vi "Signal Parameters FG.vi"(7 "Action":T1, 8 "error in (no error)":errorcluster, 10 "Signal Parameters":T2 {"Byte Order" items=["Little Endian", "Big Endian"]; "Data Type" items=["Signed", "Unsigned", "IEEE Float"]}, 11 "Device Item Ref in":T3 format="%.0x") -> (0 "error out":errorcluster, 2 "Signal Parameters":T2 {"Byte Order" items=["Little Endian", "Big Endian"]; "Data Type" items=["Signed", "Unsigned", "IEEE Float"]}, 3 "Device Item Ref out":T3=18446744073709551615 format="%.0x")   [LabVIEW 2013, in "Diagnostics Addon Shared.lvlib"]
uses:
  Diagnostics Addon Shared.lvlib
  <vilib>/NI Veristand/Custom Device API/Custom Device Item Ref.ctl
  DIDPID Signal Parameters.ctl
  FG Action.ctl
  GUID Lookup.vi
  <vilib>/NI Veristand/Custom Device API/Set Item Property (Variant).vi
  <vilib>/NI Veristand/Custom Device API/Get Item Property (Variant).vi
  <vilib>/NI Veristand/Custom Device API/Custom Device API.lvlib
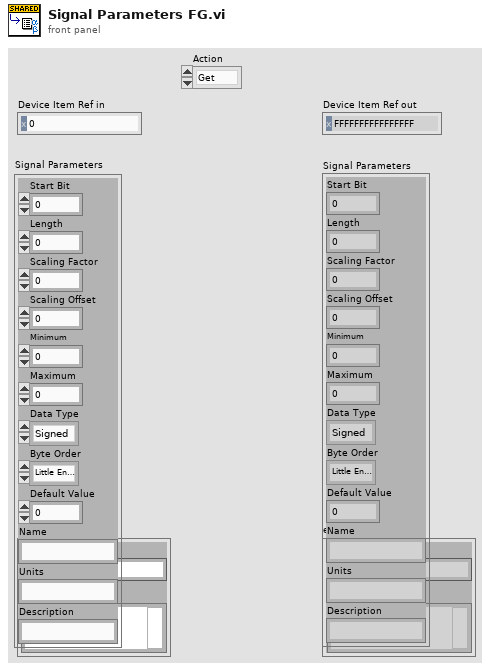
[diagram p1: front panel]
types:
  T1 = typedef "Diagnostics Addon Shared.lvlib/FG Action.ctl" = enum16{"Get", "Set"}
  T2 = typedef "Diagnostics Addon Shared.lvlib/DIDPID Signal Parameters.ctl" = cluster{"Start Bit":u8, "Length":u8, "Scaling Factor":dbl, "Scaling Offset":dbl, "Minimum":dbl, "Maximum":dbl, "Data Type":u32, "Byte Order":u32, "Default Value":dbl, "Name":string, "Units":string, "Description":string}
  T3 = typedef "Custom Device API.lvlib/Custom Device Item Ref.ctl" = u64
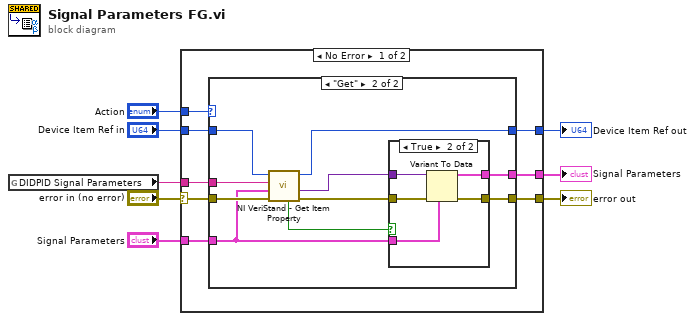
[diagram p0: block diagram]
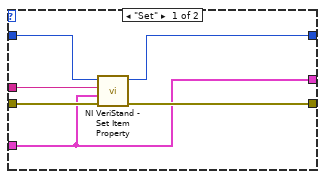
[diagram p2: hidden frame]
diagram:
  n1 = global read "GUID Lookup.vi" "DIDPID Signal Parameters"() -> (w3:string)
  n2 = case shown="No Error" "error in (no error)" {
    selector: "error in (no error)" -> [w16 w40]
    tunnel: "Device Item Ref in" -> [w15 w41]
    tunnel: [w14 w41] -> w5
    tunnel: [w13 w40] -> w6
    tunnel: [w12 _] -> w4
    tunnel: w3 -> [w11 _]
    tunnel: "Signal Parameters" -> [w10 _]
    tunnel: "Action" -> [w9 _]
    frame No Error {
      n3 = case shown="\"Get\"" w9 {
        tunnel: w16 -> [w22 w32]
        tunnel: w15 -> [w18 w31]
        tunnel: [w17 w30] -> w14
        tunnel: [w21 w28] -> w13
        tunnel: [w20 w26] -> w12
        tunnel: w11 -> [w19 w25]
        tunnel: w10 -> [w20 w24]
        frame "Set" {
          n4 = call-poly <vilib>:"NI VeriStand - Set Item Property.vi"("error in (no error)"=w22, "Value"=w20, "Property Name"=w19, "Item Ref in"=w18) -> ("error out"=w21:errorcluster, "Item Ref out"=w17:T3)  [unwired: 5 in, 1 out]
        }
        frame "Get" {
          n5 = call-poly <vilib>:"NI VeriStand - Get Item Property.vi"("error in (no error)"=w32, "Default Value"=w24, "Property Name"=w25, "Item Ref in"=w31) -> ("error out"=w29:errorcluster, "Value"=w27:variant, "Item Ref out"=w30:T3, "Found?"=w23:bool)  [unwired: 4 in]
          n6 = case shown="True" w23 {
            tunnel: w29 -> [w33 w39]
            tunnel: [w33 w38] -> w28
            tunnel: w27 -> [_ w37]
            tunnel: [w34 w36] -> w26
            tunnel: w24 -> [w34 w35]
            frame False {
            }
            frame True {
              n7 = Variant To Data(error in=w39, type=w35, Variant=w37) -> (data=w36:T2, error out=w38:errorcluster)
            }
          }
        }
      }
    }
    frame Error {
    }
  }
  "error out" <- w6
  "Device Item Ref out" <- w5
  "Signal Parameters" <- w4
